vi "Configure Memory Location.vi"(8 "error in (no error)":errorcluster, 10 "Memory Location (000)":i32 min=0 max=399 step=1 format="%03.0f", 11 "VISA resource name":refnum<visa-resource-name>) -> (0 "error out":errorcluster, 3 "VISA resource name out":refnum<visa-resource-name>)   [LabVIEW 2018, in "EFD Ultimus V.lvlib"]
doc: "This vi changes the selected memory location of the dispenser. The LCD screen will update to the new memory location, including updating the dispense time, pressure and vacuum parameter.\nHost Format: CH--ccc\nWhere\n-- :two spaces\nccc :The 3-digit memory location from 0-399. The dispenser will automatically limit the value to prevent \n any errors"
uses:
  EFD Ultimus V.lvlib
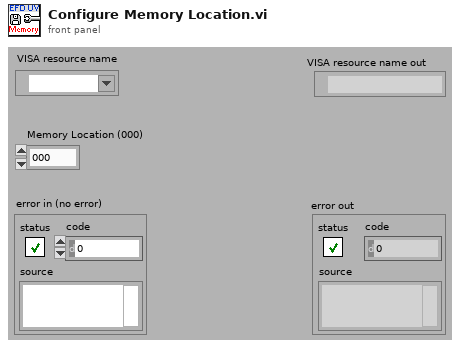
[diagram p1: front panel]
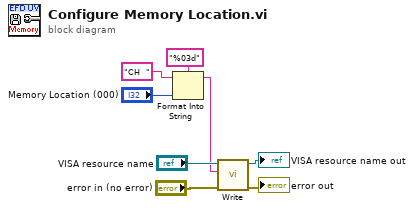
[diagram p0: block diagram]
diagram:
  n1 = Format Into String(format string="%03d", initial string="CH  " ("string"), "Memory Location (000)") -> (resulting string=w4:string)  [unwired: 1 in, 1 out]
  n2 = call "Write.vi"("error in (no error)"="error in (no error)", "Command To Write"=w4, "VISA resource name"="VISA resource name") -> ("error out"=→"error out":errorcluster, "VISA resource name out"=→"VISA resource name out":refnum<visa-resource-name>)  [unwired: 7 out]
